vi "Add Alarm.vi"(8 "error in (no error)":errorcluster, 10 "Alarm":T1, 11 "Actor in":refnum<class "Alarm Handler Actor.lvclass">) -> (0 "error out":errorcluster, 3 "Actor out":refnum<class "Alarm Handler Actor.lvclass">)   [LabVIEW 2015, in "Alarm Handler Actor.lvclass"]
doc: "Searches through the Active Alarms and adds the <b>Alarm</b> if it has not been found. Additionally it is logged.\n\nIf the <b>Alarm</b> is already active then the Count is incremented and the Last Error timestamp is updated."
uses:
  Alarm Handler Actor.lvclass
  Active Alarm.ctl
  Alarm Details.ctl
  Alarm Handler Actor.lvclass/Alarm Handler Actor.ctl
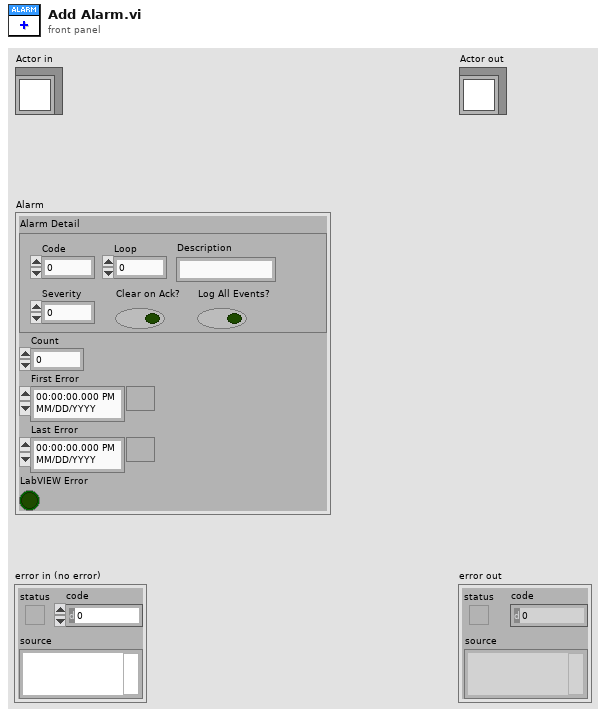
[diagram p1: front panel]
types:
  T1 = typedef "Alarm Handler Actor.lvclass/Active Alarm.ctl" = cluster{"Alarm Detail":T2, "Count":i32, "First Error":timestamp, "Last Error":timestamp, "LabVIEW Error":bool}
  T2 = typedef "Alarm Handler Actor.lvclass/Alarm Details.ctl" = cluster{"Code":i32, "Loop":i32, "Description":string, "Severity":i32, "Clear on Ack?":bool, "Log All Events?":bool}
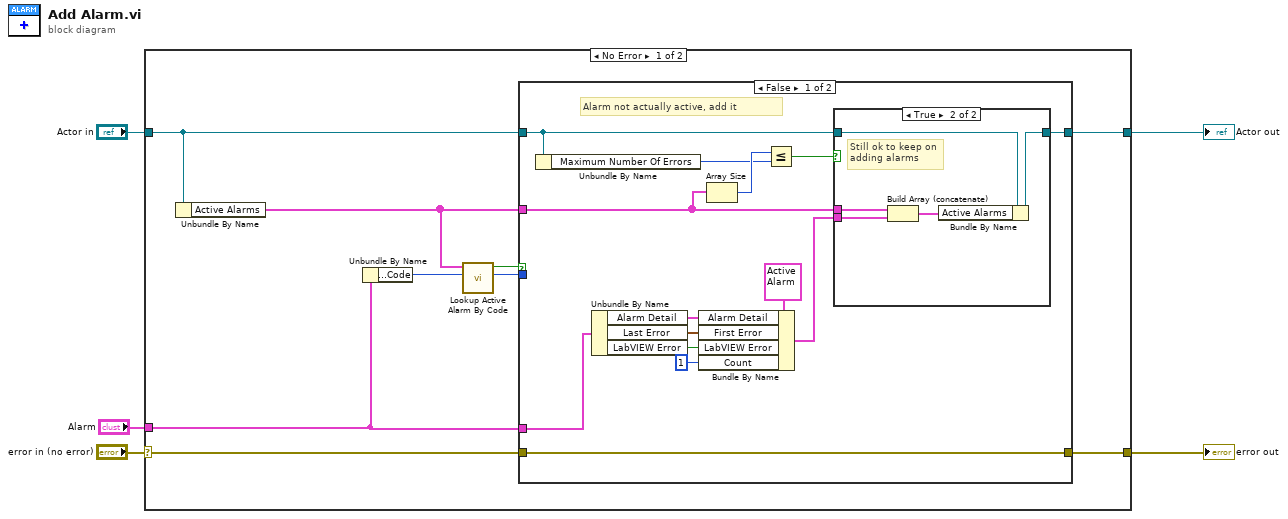
[diagram p0: block diagram]
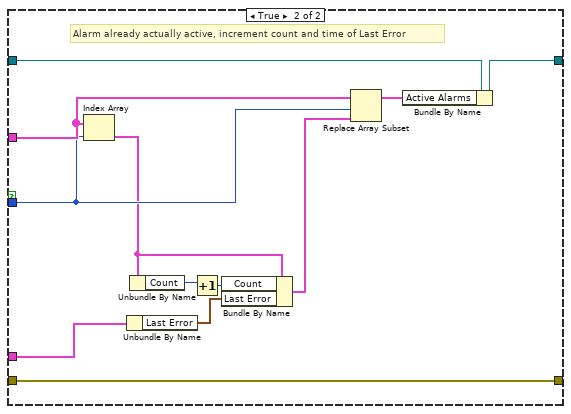
[diagram p3: hidden frame]
diagram:
  n1 = case shown="No Error" "error in (no error)" {
    selector: "error in (no error)" -> [w7 w48]
    tunnel: [w6 w48] -> w4
    tunnel: [w13 w47] -> w2
    tunnel: "Actor in" -> [w14 w47]
    tunnel: "Alarm" -> [w8 _]
    frame No Error {
      n2 = Unbundle By Name(w14) -> ("Active Alarms"=w10:T1[])
      n3 = Unbundle By Name(w8) -> ("Alarm Detail.Code"=w12:i32)
      n4 = call "Lookup Active Alarm By Code.vi"("Code"=w12, "Active Alarms"=w10) -> ("Index"=w9:i32, "Found"=w11:bool)  [unwired: 8 in]
      n5 = case shown="False" w11 {
        tunnel: w14 -> [w21 w46]
        tunnel: [w22 w45] -> w13
        tunnel: w10 -> [w20 w44]
        tunnel: w9 -> [_ w40]
        tunnel: w8 -> [w16 w37]
        tunnel: w7 -> [w15 w35]
        tunnel: [w15 w35] -> w6
        frame False {
          # "Alarm not actually active, add it"
          n6 = Unbundle By Name(w21) -> ("Maximum Number Of Errors"=w18:i32)
          n7 = Unbundle By Name(w16) -> ("Alarm Detail"=w26:T2, "Last Error"=w27:timestamp, "LabVIEW Error"=w28:bool)
          n8 = Bundle By Name(cluster=T1 {"Alarm Detail"={"Code"=0, "Loop"=0, "Description"="", "Severity"=0, "Clear on Ack?"=FALSE, "Log All Events?"=FALSE}, "Count"=0, "First Error"=timestamp(0 s since 1904-01-01), "Last Error"=timestamp(0 s since 1904-01-01), "LabVIEW Error"=FALSE} ("Present Errors"), "Alarm Detail"=w26, "First Error"=w27, "LabVIEW Error"=w28, "Count"=1) -> (w23:T1)
          n9 = Array Size(array=w20) -> (size(s)=w19:i32)
          n10 = Less Or Equal?(x=w19, y=w18) -> (x <= y?=w17:bool)
          n11 = case shown="True" w17 {
            tunnel: w20 -> [_ w34]
            tunnel: w23 -> [_ w33]
            tunnel: [w29 w30] -> w22
            tunnel: w21 -> [w29 w31]
            frame False {
              # "Do not continue to allocate memory for alarms unbounded.\nDesirable to keep oldest alarms so just discard and new ones that are generated"
            }
            frame True {
              # "Still ok to keep on adding alarms"
              n12 = Build Array (concatenate)(w34, w33) -> (w32:T1[])
              n13 = Bundle By Name(cluster=w31, "Active Alarms"=w32) -> (w30:refnum<class "Alarm Handler Actor.lvclass">)
            }
          }
        }
        frame True {
          # "Alarm already actually active, increment count and time of Last Error"
          n14 = Index Array(array=w44, index=w40) -> (element=w39:T1)
          n15 = Unbundle By Name(w37) -> ("Last Error"=w36:timestamp)
          n16 = Unbundle By Name(w39) -> ("Count"=w42:i32)
          n17 = Increment(x=w42) -> (x+1=w43:i32)
          n18 = Bundle By Name(cluster=w39, "Count"=w43, "Last Error"=w36) -> (w38:T1)
          n19 = Replace Array Subset(array=w44, new element=w38, index=w40) -> (w41:T1[])
          n20 = Bundle By Name(cluster=w46, "Active Alarms"=w41) -> (w45:refnum<class "Alarm Handler Actor.lvclass">)
        }
      }
    }
    frame Error {
    }
  }
  "error out" <- w4
  "Actor out" <- w2
